vi "flowtestloop.vi"() -> ()   [LabVIEW 2015]
uses:
  <vilib>/Instr/_visa.llb/VISA Configure Serial Port (Instr).vi
panel:
  out "data report":string
  out "Sent Byte Array":u8[](array[numeric])
  in  "Measurement Options":T1(ring)
  out "Returned Byte Array":u8[](array[numeric])
  out "byte count":u32
  out "error out":errorcluster
  in  "error in (no error)":errorcluster
  out "String returned":string
  out "String written":string
  in  "VISA Configure or Open?":enum16{"Open", "Configure"}(ring)=enum."Configure"
  in  "VISA resource name":refnum<visa-resource-name>
  in  "Control Options":T2(ring)
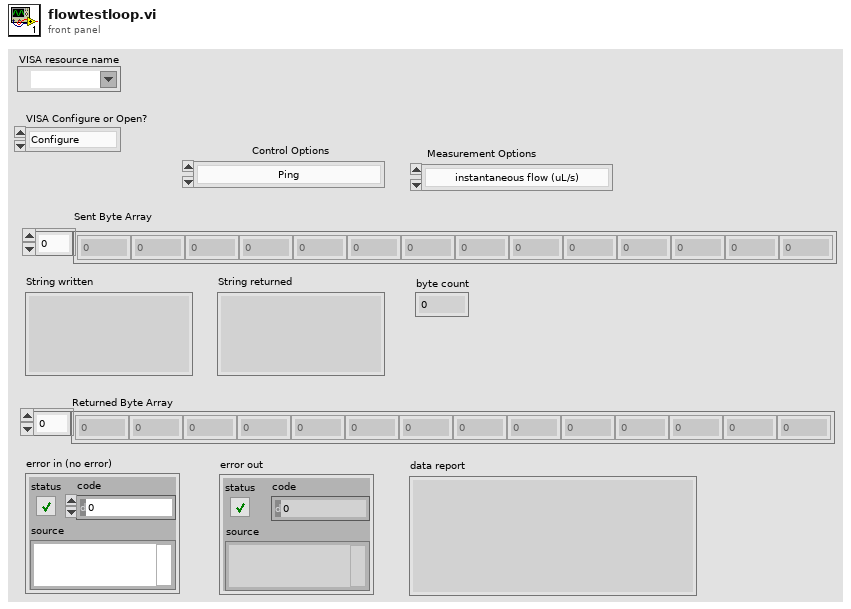
[diagram p1: front panel]
types:
  T1 = enum16{"instantaneous flow (uL/s)", "temperature (C)", "accumulated volume (uL)", "current output (mA)", "freq output (kHz)"}
  T2 = enum16{"Ping", "Restart", "Get Values", "Get Identity"}
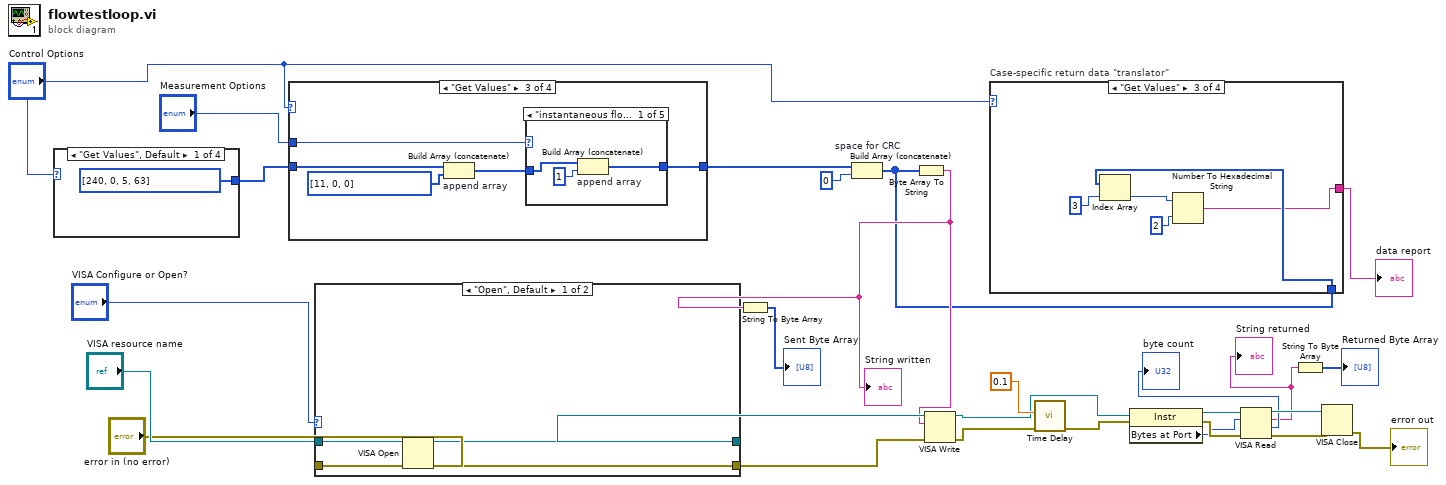
[diagram p0: block diagram]
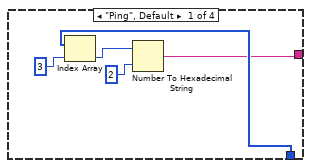
[diagram p2: hidden frame]
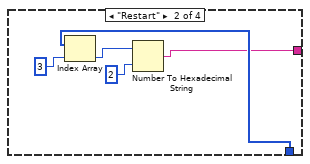
[diagram p3: hidden frame]
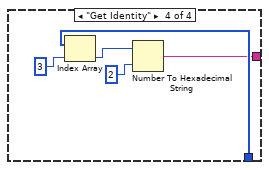
[diagram p4: hidden frame]
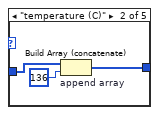
[diagram p7: hidden frame]
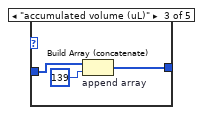
[diagram p8: hidden frame]
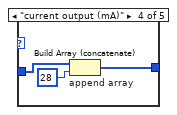
[diagram p9: hidden frame]
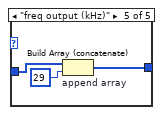
[diagram p10: hidden frame]
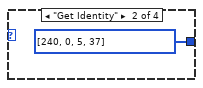
[diagram p12: hidden frame]
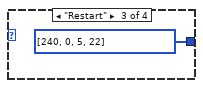
[diagram p13: hidden frame]
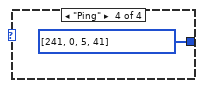
[diagram p14: hidden frame]
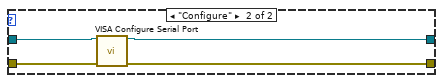
[diagram p15: hidden frame]
diagram:
  n1 = case shown="\"Get Values\", Default" "Control Options" {
    tunnel: [u8[] [240, 0, 5, 63] ("unsigned byte array") u8[] [240, 0, 5, 37] ("unsigned byte array") u8[] [240, 0, 5, 22] ("unsigned byte array") u8[] [241, 0, 5, 41]] -> w11
    frame "Get Values", Default {
    }
    frame "Get Identity" {
    }
    frame "Restart" {
    }
    frame "Ping" {
    }
  }
  n2 = case shown="\"Get Values\"" "Control Options" {
    tunnel: [w32 w33 w34 w54] -> w9
    tunnel: w11 -> [w32 w33 w38 w54]
    tunnel: "Measurement Options" -> [_ _ w36 _]
    frame "Ping", Default {
    }
    frame "Restart" {
    }
    frame "Get Values" {
      n3 = Build Array (concatenate) "append array"(w38, u8[] [11, 0, 0]) -> (w35:u8[])
      n4 = case shown="\"instantaneous flow (uL/s)\", Default" w36 {
        tunnel: w35 -> [w40 w44 w46 w49 w52]
        tunnel: [w39 w43 w45 w48 w51] -> w34
        frame "instantaneous flow (uL/s)", Default {
          n5 = Build Array (concatenate) "append array"(w40, u8 1) -> (w39:u8[])
        }
        frame "temperature (C)" {
          n6 = Build Array (concatenate) "append array"(w44, u8 136) -> (w43:u8[])
        }
        frame "accumulated volume (uL)" {
          n7 = Build Array (concatenate) "append array"(w46, u8 139) -> (w45:u8[])
        }
        frame "current output (mA)" {
          n8 = Build Array (concatenate) "append array"(w49, u8 28) -> (w48:u8[])
        }
        frame "freq output (kHz)" {
          n9 = Build Array (concatenate) "append array"(w52, u8 29) -> (w51:u8[])
        }
      }
    }
    frame "Get Identity" {
    }
  }
  n10 = case shown="\"Open\", Default" "VISA Configure or Open?" {
    tunnel: "VISA resource name" -> [w58 w62]
    tunnel: [w57 w61] -> w24
    tunnel: "error in (no error)" -> [w56 w60]
    tunnel: [w55 w59] -> w21
    frame "Open", Default {
      n11 = VISA Open(error in (no error)=w56, VISA resource name=w58) -> (VISA resource name=w57:refnum<visa-resource-name>, error out=w55:errorcluster)  [unwired: 3 in]
    }
    frame "Configure" {
      n12 = call-poly "VISA Configure Serial Port"("VISA resource name"=w62, "error in (no error)"=w60) -> ("VISA resource name out"=w61:refnum<visa-resource-name>, "error out"=w59:errorcluster)  [unwired: 12 in]
    }
  }
  n13 = Build Array (concatenate) "space for CRC"(w9, u8 0) -> (w2:u8[])
  n14 = Byte Array To String(unsigned byte array=w2) -> (string=w8:string)
  "String written" <- w8
  n15 = String To Byte Array(string=w8) -> (unsigned byte array=→"Sent Byte Array":u8[])
  n16 = VISA Write(VISA resource name=w24, write buffer=w8, error in (no error)=w21) -> (VISA resource name out=w18:refnum<visa-resource-name>, error out=w20:errorcluster)  [unwired: 1 out]
  n17 = case "Case-specific return data \"translator\"" shown="\"Get Values\"" "Control Options" {
    tunnel: w2 -> [w64 w69 w76 w79]
    tunnel: [w63 w68 w73 w78] -> w1
    frame "Ping", Default {
      n18 = Index Array(array=w64, index=3) -> (element=w67:u8)
      n19 = Number To Hexadecimal String(1:2, 2:w67) -> (0:w63:string)
    }
    frame "Restart" {
      n20 = Index Array(array=w69, index=3) -> (element=w72:u8)
      n21 = Number To Hexadecimal String(1:2, 2:w72) -> (0:w68:string)
    }
    frame "Get Values" {
      n22 = Index Array(array=w76, index=3) -> (element=w75:u8)
      n23 = Number To Hexadecimal String(1:2, 2:w75) -> (0:w73:string)
    }
    frame "Get Identity" {
      n24 = Index Array(array=w79, index=3) -> (element=w82:u8)
      n25 = Number To Hexadecimal String(1:2, 2:w82) -> (0:w78:string)
    }
  }
  "data report" <- w1
  n26 = call "Time Delay"("error in (no error)"=w20, "Delay Time (s)"=0.1) -> ("error out"=w17:errorcluster)  [unwired: 9 in]
  n27 = property class="Instr"(reference=w18, error in=w17) -> (reference out=w16:refnum<visa-resource-name>, error out=w15:errorcluster, "Bytes at Port"=w14:u32)
  n28 = VISA Read(VISA resource name=w16, byte count=w14, error in (no error)=w15) -> (VISA resource name out=w23:refnum<visa-resource-name>, read buffer=w6:string, return count=→"byte count":u32, error out=w19:errorcluster)
  "String returned" <- w6
  n29 = String To Byte Array(string=w6) -> (unsigned byte array=→"Returned Byte Array":u8[])
  n30 = VISA Close(VISA resource name=w23, error in (no error)=w19) -> (error out=→"error out":errorcluster)
